vi "System Explorer - Add content to System Explorer library.vi"(8 "error in (no error)":errorcluster, 11 "CD Wizard - Internal Data IN":T1) -> (0 "error out":errorcluster)   [LabVIEW 2015]
doc: "Add all virtual folders and VIs to the System Explorer library."
uses:
  TypDef/CD Wizard - Internal data.ctl
  TypDef/CD Wizard - Execution Mode.ctl
  TypDef/CD Wizard - Extra Page Name and GUID.ctl
  Constants/Constants TypDef/CD System Explorer lvlib.ctl
  TypDef/Add Item - Type.ctl
  Constants/CD System Explorer lvlib.vi
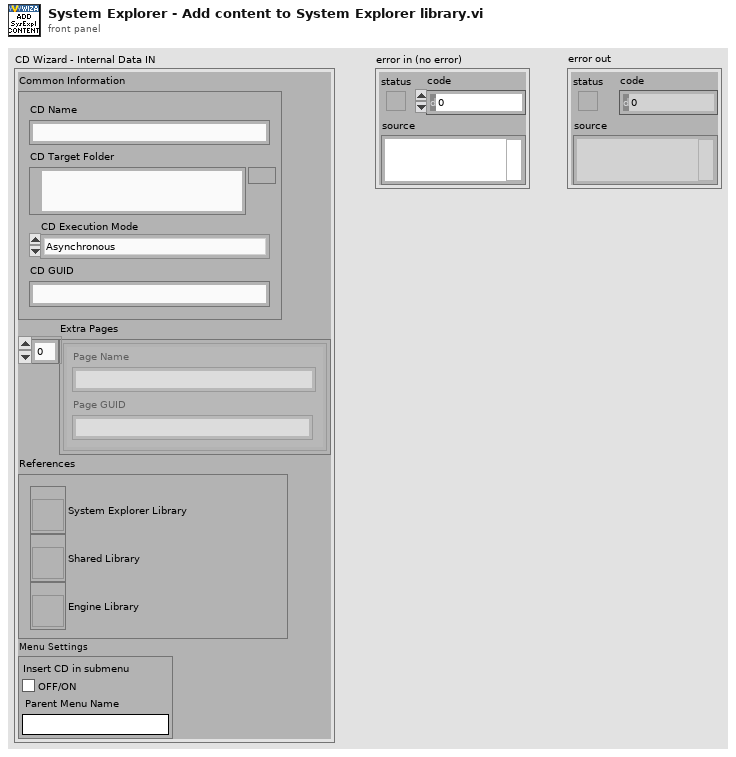
[diagram p1: front panel]
types:
  T1 = typedef "CD Wizard - Internal data.ctl" = cluster{"Common Information":cluster{"CD Name":string, "CD Target Folder":path, "CD Execution Mode":T2, "CD GUID":string}, "Extra Pages":T3[], "References":cluster{"System Explorer Library":refnum<vi>, "Shared Library":refnum<vi>, "Engine Library":refnum<vi>}, "Menu Settings":cluster{"Insert CD in submenu":bool, "Parent Menu Name":string}}
  T2 = typedef "CD Wizard - Execution Mode.ctl" = enum16{"Asynchronous", "Inline HW Interface", "Inline Model Interface", "Inline Timing and Sync", "Asynchronous Timing and Sync"}
  T3 = typedef "CD Wizard - Extra Page Name and GUID.ctl" = cluster{"Page Name":string, "Page GUID":string}
  T4 = typedef "CD System Explorer lvlib.ctl" = enum16{"LibraryFileName", "LibraryFolderName", "System Explorer.FolderName", "System Explorer.Dynamically Called.FolderName", "System Explorer.Dynamically Called.Extra Pages.FolderName", "System Explorer.Dynamically Called.Extra Pages.TemplatePathAndName", "System Explorer.Dynamically Called.Main Page.VIName", "System Explorer.Dynamically Called.Main Page.TemplatePathAndName", "System Explorer.Dynamically Called.Initialization VI.VIName", "System Explorer.Dynamically Called.Initialization VI.TemplatePathAndName", "System Explorer.SubVI.FolderName", "System Explorer.Types.FolderName"}
  T5 = typedef "Add Item - Type.ctl" = string
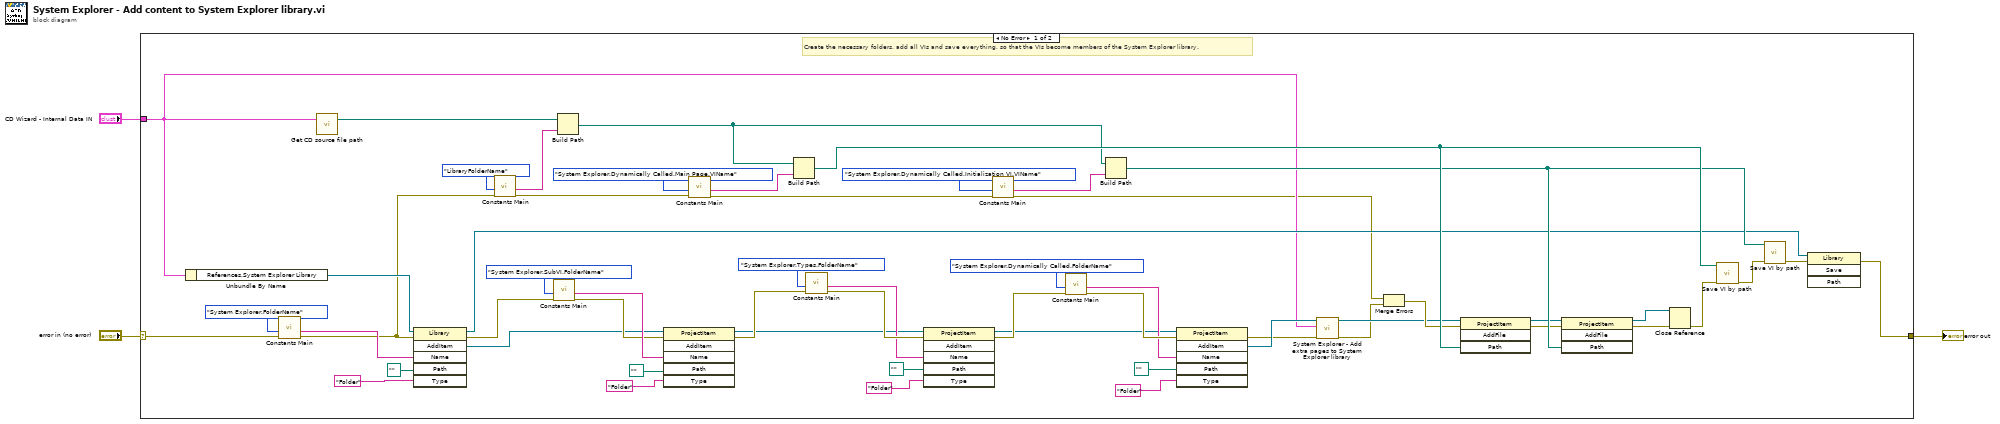
[diagram p0: block diagram]
diagram:
  n1 = case shown="No Error" "error in (no error)" {
    selector: "error in (no error)" -> [w59 w60]
    tunnel: "CD Wizard - Internal Data IN" -> [w11 _]
    tunnel: [w58 w60] -> w1
    frame No Error {
      # "Create the necessary folders, add all VIs and save everything, so that the VIs become members of the System Explorer library."
      n2 = Unbundle By Name(w11) -> ("References.System Explorer Library"=w17:refnum<vi>)
      n3 = call-poly "Constants Main.vi"("error in (no error)"=w59, "Action"=CD_System_Explorer_lvlib."System Explorer.FolderName") -> ("error out"=w5:errorcluster, "Output"=w54:string)  [unwired: 8 in]
      n4 = call "Get CD source file path.vi"("CD Wizard - Internal Data"=w11) -> ("CD Source file path"=w16:path)  [unwired: 2 in]
      n5 = invoke class="Library" method="AddItem"(reference=w17, error in=w5, "Name"=w54, "Path"=path "", "Type"=T5 "Folder" ("Add Item - Type")) -> (reference out=w19:refnum<vi>, error out=w31:errorcluster, "AddItem"=w18:refnum<vi>)  [unwired: 1 in, 3 out]
      n6 = call-poly "Constants Main.vi"("error in (no error)"=w5, "Action"=CD_System_Explorer_lvlib."LibraryFolderName") -> ("error out"=w6:errorcluster, "Output"=w4:string)  [unwired: 8 in]
      n7 = call-poly "Constants Main.vi"("error in (no error)"=w31, "Action"=CD_System_Explorer_lvlib."System Explorer.SubVI.FolderName") -> ("error out"=w39:errorcluster, "Output"=w41:string)  [unwired: 8 in]
      n8 = Build Path(base path=w16, name or relative path=w4) -> (appended path=w8:path)
      n9 = invoke class="ProjectItem" method="AddItem"(reference=w18, error in=w39, "Name"=w41, "Path"=path "", "Type"=T5 "Folder" ("Add Item - Type")) -> (reference out=w23:refnum<vi>, error out=w30:errorcluster)  [unwired: 1 in, 4 out]
      n10 = call-poly "Constants Main.vi"("error in (no error)"=w6, "Action"=CD_System_Explorer_lvlib."System Explorer.Dynamically Called.Main Page.VIName") -> ("error out"=w10:errorcluster, "Output"=w52:string)  [unwired: 8 in]
      n11 = Build Path(base path=w8, name or relative path=w52) -> (appended path=w45:path)
      n12 = call-poly "Constants Main.vi"("error in (no error)"=w30, "Action"=CD_System_Explorer_lvlib."System Explorer.Types.FolderName") -> ("error out"=w36:errorcluster, "Output"=w34:string)  [unwired: 8 in]
      n13 = invoke class="ProjectItem" method="AddItem"(reference=w23, error in=w36, "Name"=w34, "Path"=path "", "Type"=T5 "Folder" ("Add Item - Type")) -> (reference out=w21:refnum<vi>, error out=w22:errorcluster)  [unwired: 1 in, 4 out]
      n14 = call-poly "Constants Main.vi"("error in (no error)"=w10, "Action"=CD_System_Explorer_lvlib."System Explorer.Dynamically Called.Initialization VI.VIName") -> ("error out"=w9:errorcluster, "Output"=w51:string)  [unwired: 8 in]
      n15 = call-poly "Constants Main.vi"("error in (no error)"=w22, "Action"=CD_System_Explorer_lvlib."System Explorer.Dynamically Called.FolderName") -> ("error out"=w28:errorcluster, "Output"=w26:string)  [unwired: 8 in]
      n16 = Build Path(base path=w8, name or relative path=w51) -> (appended path=w44:path)
      n17 = invoke class="ProjectItem" method="AddItem"(reference=w21, error in=w28, "Name"=w26, "Path"=path "", "Type"=T5 "Folder" ("Add Item - Type")) -> (error out=w13:errorcluster, "AddItem"=w15:refnum<vi>)  [unwired: 1 in, 4 out]
      n18 = call "System Explorer - Add extra pages to System Explorer library.vi"("error in (no error)"=w13, "CD Wizard - Internal Data"=w11, "ProjectItem IN"=w15) -> ("error out"=w12:errorcluster, "ProjectItem OUT"=w14:refnum<vi>)  [unwired: 7 in]
      n19 = Merge Errors(w9, w12) -> (w20:errorcluster)
      n20 = invoke class="ProjectItem" method="AddFile"(reference=w14, error in=w20, "Path"=w45) -> (reference out=w24:refnum<vi>, error out=w25:errorcluster)  [unwired: 1 in, 2 out]
      n21 = invoke class="ProjectItem" method="AddFile"(reference=w24, error in=w25, "Path"=w44) -> (reference out=w42:refnum<vi>, error out=w48:errorcluster)  [unwired: 1 in, 2 out]
      n22 = Close Reference(reference=w42, error in (no error)=w48) -> (error out=w49:errorcluster)
      n23 = call "Save VI by path.vi"("error in (no error)"=w49, "VI path"=w45) -> ("error out"=w47:errorcluster)  [unwired: 9 in]
      n24 = call "Save VI by path.vi"("error in (no error)"=w47, "VI path"=w44) -> ("error out"=w46:errorcluster)  [unwired: 9 in]
      n25 = invoke class="Library" method="Save"(reference=w19, error in=w46) -> (error out=w58:errorcluster)  [unwired: 2 in, 3 out]
    }
    frame Error {
      # "Output default values."
    }
  }
  "error out" <- w1
